vi "GetNpoint_andVector.vi"(9 "max":dbl, 10 "step":dbl, 11 "min":dbl) -> (1 "Point Array":dbl[](array[numeric]), 3 "Npoints":dbl)   [LabVIEW 2018, in "Sequences.lvlib"]
uses:
  Sequences.lvlib
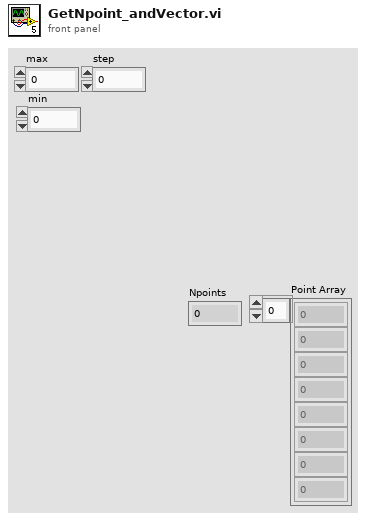
[diagram p1: front panel]
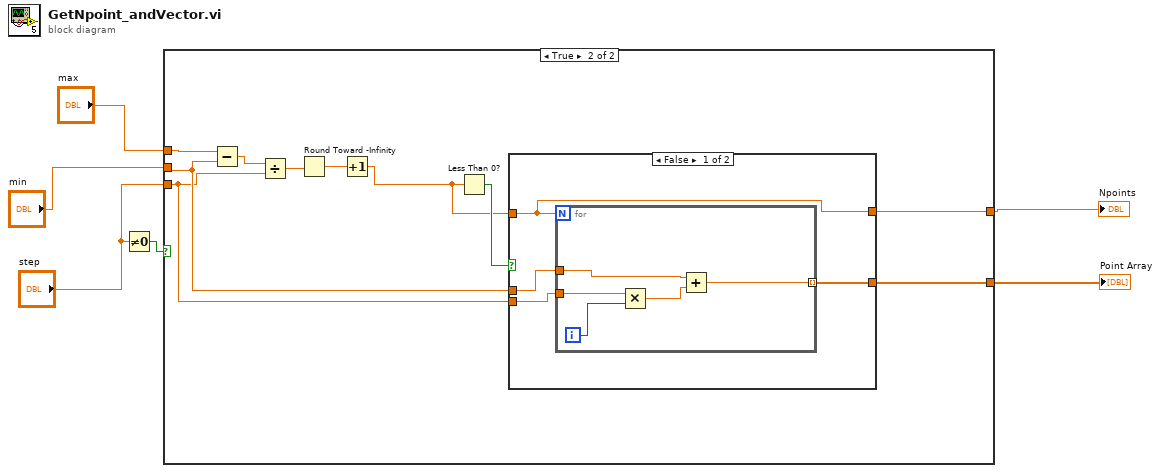
[diagram p0: block diagram]
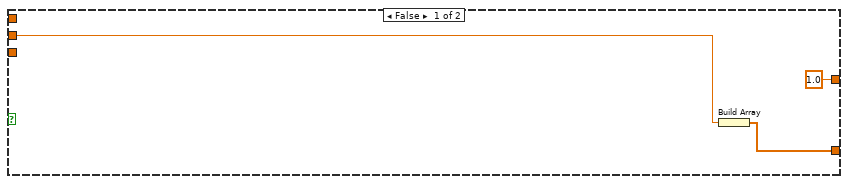
[diagram p2: hidden frame]
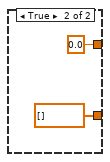
[diagram p3: hidden frame]
diagram:
  n1 = Not Equal To 0?(x="step") -> (x != 0?=w4:bool)
  n2 = case shown="True" w4 {
    tunnel: "max" -> [_ w19]
    tunnel: "min" -> [w8 w15]
    tunnel: "step" -> [_ w14]
    tunnel: [w7 w13] -> w6
    tunnel: [1.0 w12] -> w5
    frame False {
      n3 = Build Array(w8) -> (w7:dbl[])
    }
    frame True {
      n4 = Subtract(x=w19, y=w15) -> (x-y=w18:dbl)
      n5 = Divide(x=w18, y=w14) -> (x/y=w17:dbl)
      n6 = Round Toward -Infinity(1:w17) -> (0:w11:dbl)
      n7 = Increment(x=w11) -> (x+1=w10:dbl)
      n8 = Less Than 0?(x=w10) -> (x < 0?=w16:bool)
      n9 = case shown="False" w16 {
        tunnel: w10 -> [w20 _]
        tunnel: w15 -> [w23 _]
        tunnel: w14 -> [w22 _]
        tunnel: [w21 dbl[] []] -> w13
        tunnel: [w20 0.0] -> w12
        frame False {
          n10 = for {
            N: w20 -> [_]
            tunnel: w23 -> [w25]
            tunnel: w22 -> [w28]
            tunnel: [w24] -> w21 mode=indexing
            i -> [w27]
            n11 = Multiply(x=w28, y=w27) -> (x*y=w26:dbl)
            n12 = Add(x=w25, y=w26) -> (x+y=w24:dbl)
          }
        }
        frame True {
        }
      }
    }
  }
  "Point Array" <- w6
  "Npoints" <- w5
